vi "Std_Bus_Close_System.vi"(0 "ILabVIEW In":refnum<k24>) -> (19 "error out":errorcluster)   [LabVIEW 2018]
doc: "Terminates communicaiton with the <B>Watlow EZ-Zone</B> Product. This should be called once at the end of the applicaition.\n\nThis VI Driver set supports the following communication protocols. The user will select the type from the <B> InterfaceType</B> Control. There is a wait period after the port is closed to insure that any write commands initiated have proper time to complete. This time varies depending on the Interface type.\n\n<B>Serial</B> - RS 485 Communications - 0.5 second wait period.\n<B> USB </B> - USB - 1.5 second wait period.\n<B> Ethernet</B> - 4.5 second wait period."
uses:
  C:/RageATE/Instruments/Ess Temp Plate/LabView Driver/Public/Watbus.dll
  Watbus.dll
panel:
  # "Std Bus Close System"
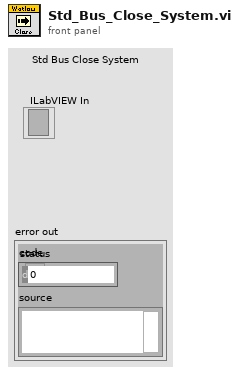
[diagram p1: front panel]
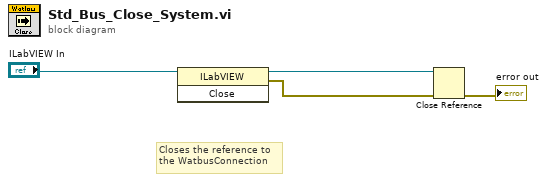
[diagram p0: block diagram]
diagram:
  # "Closes the reference to\nthe WatbusConnection"
  n1 = invoke class="ILabVIEW" method="Close"(reference="ILabVIEW In") -> (reference out=w3:refnum<k24>, error out=w2:errorcluster)  [unwired: 2 in, 1 out]
  n2 = Close Reference(reference=w3, error in (no error)=w2) -> (error out=→"error out":errorcluster)
